vi "AES-KeyExpansion.vi"(8 "error in (no error)":errorcluster, 11 "Key In":u8[](array[numeric]) format="%.0x") -> (0 "error out":errorcluster, 3 "Expanded Key [U8]":u8[](array[numeric]) format="%02x")   [LabVIEW 2020, in "Encryption.lvlib"]
doc: "Expands a Key using AES Key expansion.\n\n(c) Ton Plomp, 2011\nTHIS SOFTWARE IS PROVIDED AS IS, AND ANY WARRANTY IS REJECTED"
uses:
  Encryption.lvlib
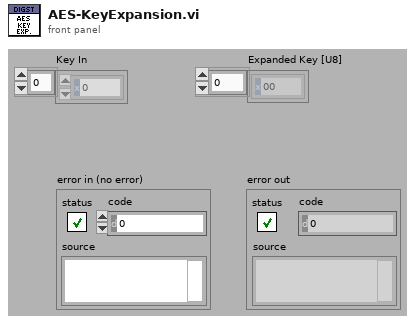
[diagram p1: front panel]
types:
  T1 = cluster{bool, i32, "String to Prepend to source (\"\")":string}
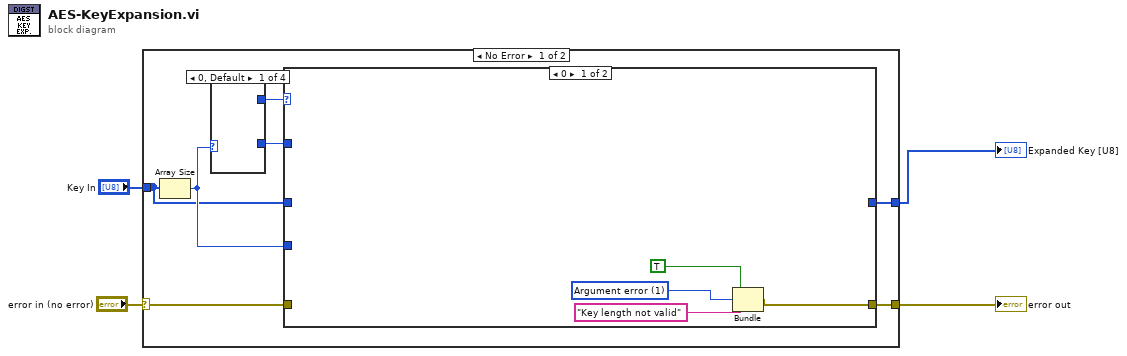
[diagram p0: block diagram]
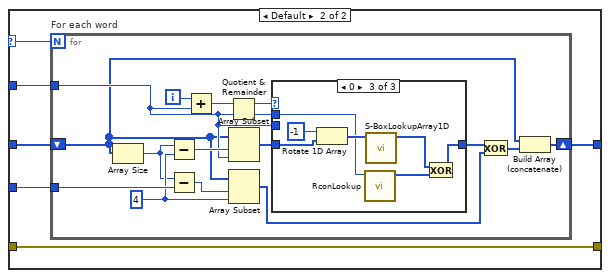
[diagram p2: hidden frame]
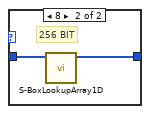
[diagram p5: hidden frame]
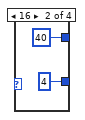
[diagram p6: hidden frame]
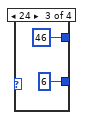
[diagram p7: hidden frame]
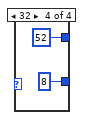
[diagram p8: hidden frame]
diagram:
  n1 = case shown="No Error" "error in (no error)" {
    selector: "error in (no error)" -> [w6 w58]
    tunnel: [w9 _] -> w4
    tunnel: "Key In" -> [w5 _]
    tunnel: [w7 w58] -> w2
    frame No Error {
      n2 = Array Size(array=w5) -> (size(s)=w11:i32)
      n3 = case shown="0, Default" w11 {
        tunnel: [_ 40 46 52] -> w8
        tunnel: [_ 4 6 8] -> w10
        frame 0, Default {
        }
        frame 16 {
        }
        frame 24 {
        }
        frame 32 {
        }
      }
      n4 = case shown="0" w8 {
        selector: w8 -> [_ w16]
        tunnel: w11 -> [_ w21]
        tunnel: w10 -> [_ w20]
        tunnel: [_ w19] -> w9
        tunnel: w5 -> [_ w18]
        tunnel: w6 -> [_ w17]
        tunnel: [w15 w17] -> w7
        frame 0 {
          w13 = 1 items=["No error", "Argument error", "Memory is full", "Out of zone", "End of file", "File already open", "Generic file I/O error", "File not found", "File permission error", "Disk is full", "Duplicate path", "Too many files open", "System feature not enabled", "Resource file not found", "Cannot add resource", "Resource not found", "Image not found", "Image memory error", "Pen does not exist", "Config type invalid", "Config token not found", "Config parse error", "Config memory error", "Bad external code format", "Bad external code offset", "External code not present", "Null window", "Destroy window error", "Null menu", "Print aborted", "Bad print record", "Print driver error", "Windows error during printing", "Memory error during printing", "Print dialog error", "Generic print error", "Invalid device refnum", "Device not found", "Device parameter error", "Device unit error", "Cannot open device", "Device call aborted", "Generic error", "Cancelled by user", "Object ID too low", "Object ID too high", "Object not in heap", "Unknown heap", "Unknown object (invalid DefProc)", "Unknown object (DefProc not in table)", "Message out of range", "Invalid (null) method", "Unknown message", "Manager call not supported", "Bad address", "Network operation in progress", "Network operation timed out", "Connection is busy", "Network attribute not supported", "Network error", "Address in use", "System out of memory", "Connection aborted", "Connection refused", "Not connected", "Already connected", "Connection closed", "Initialization error (interapplication manager)", "Bad occurrence", "Wait on unbound occurrence handler", "Occurrence queue overflow", "Datalog type conflict", "Unused", "Unrecognized type (interapplication manager)", "Memory corrupt", "Failed to make temporary DLL", "Old CIN version", "Drag socket not found", "Failed to load drop-object", "Failed to register OLE object", "Failed to release OLE object", "Format specifier type mismatch", "Unknown format specifier", "Too few format specifiers", "Too many format specifiers", "Scan failed", "Newer CIN version", "Error converting to variant", "Runtime menu error", "Password tampered", "Variant attribute not found", "Incompatible variant data type", "Event data is not available", "Event Store is not present", "Occurrence is not found", "Event Queue is not created", "Event info is not available", "Refnum passed is NULL", "Error retrieving Class GUID", "Error retrieving CoClass GUID", "Error retrieving TypeLib GUID.", "Bad built application magic bytes.", "Specific driver is different from the specific driver associated with the Logical Name.", "There is no session opened to the class driver.", "Max Error", "MAX - Error with config objects", "MAX - Error loading configuration", "MAX - Group not supported"]
          n5 = Bundle(TRUE, w13, "String to Prepend to source (\"\")"="Key length not valid" ("String to Prepend to source (\"\")")) -> (w15:T1)  [unwired: 1 in]
        }
        frame Default {
          n6 = for "For each word" {
            N: w16 -> [_]
            shift-right: [w37] -> w19
            shift-left: w18 -> [w24]
            tunnel: w21 -> [w36]
            tunnel: w20 -> [w25]
            i -> [w33]
            w28 = 4 ("y")
            n7 = Array Size(array=w24) -> (size(s)=w22:i32)
            n8 = Subtract(x=w22, y=w28) -> (x-y=w35:i32)
            n9 = Subtract(x=w22, y=w36) -> (x-y=w23:i32)
            n10 = Add(x=w33, y=w25) -> (x+y=w29:i32)
            n11 = Quotient & Remainder(x=w29, y=w25) -> (x-y*floor(x/y)=w34:i32, floor(x/y)=w26:i32)
            n12 = Array Subset(array=w24, index=w35, length=w25) -> (w30:u8[])
            n13 = Array Subset(array=w24, index=w23, length=w28) -> (w32:u8[])
            n14 = case shown="0" w34 {
              tunnel: w30 -> [w38 w39 w50]
              tunnel: [w38 w40 w45] -> w31
              tunnel: w25 -> [_ w41 _]
              tunnel: w26 -> [_ _ w46]
              frame Default {
              }
              frame 4 {
                n15 = case shown="Default" w41 {
                  tunnel: [w42 w43] -> w40
                  tunnel: w39 -> [w42 w44]
                  frame Default {
                  }
                  frame 8 {
                    # "256 BIT"
                    n16 = call "S-BoxLookupArray1D.vi"("In"=w44) -> ("Out"=w43:u8[])  [unwired: 10 in]
                  }
                }
              }
              frame 0 {
                n17 = Rotate 1D Array(1:w50, 2:-1 ("n")) -> (0:w48:u8[])
                n18 = call "RconLookup.vi"("iteration"=w46) -> ("LookUp-Out"=w49:u8[])  [unwired: 10 in]
                n19 = call "S-BoxLookupArray1D.vi"("In"=w48) -> ("Out"=w47:u8[])  [unwired: 10 in]
                n20 = Exclusive Or(1:w49, 2:w47) -> (0:w45:u8[])
              }
            }
            n21 = Exclusive Or(1:w32, 2:w31) -> (0:w27:u8[])
            n22 = Build Array (concatenate)(w24, w27) -> (w37:u8[])
          }
        }
      }
    }
    frame Error {
    }
  }
  "Expanded Key [U8]" <- w4
  "error out" <- w2
